vi "FGV_DataPackerParentVI.vi"(7 "Enum":T1, 10 "Callers (Main VI name)":string, 11 "This Computer Name":string) -> (2 "Parent VI to the DataPacker Daemon (Main VI name)":string, 3 "This Computer Name":string)   [LabVIEW 2018, in "feGEM DataPacker.lvlib"]
uses:
  Set_And_Get_Enum.ctl
  feGEM DataPacker.lvlib
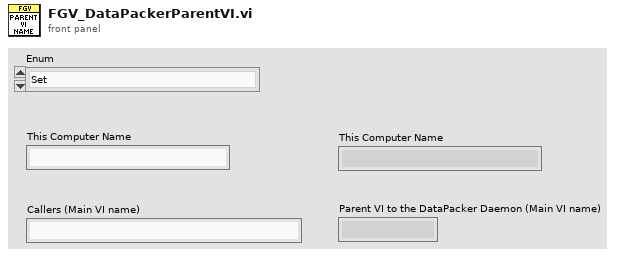
[diagram p1: front panel]
types:
  T1 = typedef "feGEM DataPacker.lvlib/Set_And_Get_Enum.ctl" = enum16{"Set", "Get"}
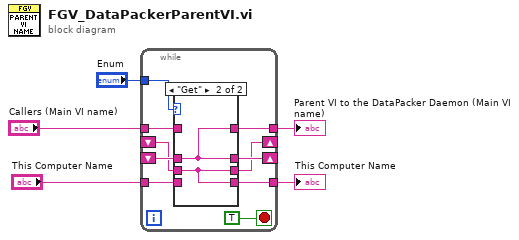
[diagram p0: block diagram]
diagram:
  n1 = while {
    tunnel: "Enum" -> [w15]
    tunnel: "Callers (Main VI name)" -> [w14]
    tunnel: [w13] -> w1
    shift-right: [w12] -> _
    shift-left: _ -> [w11]
    tunnel: "This Computer Name" -> [w9]
    tunnel: [w10] -> w2
    shift-right: [w8] -> _
    shift-left: _ -> [w7]
    stop <- TRUE stop-if-true
    n2 = case shown="\"Get\"" w15 {
      tunnel: w14 -> [w17 _]
      tunnel: [w17 w19] -> w13
      tunnel: [w17 w19] -> w12
      tunnel: w11 -> [_ w19]
      tunnel: [w16 w18] -> w10
      tunnel: w9 -> [w16 _]
      tunnel: [w16 w18] -> w8
      tunnel: w7 -> [_ w18]
      frame "Set", Default {
      }
      frame "Get" {
      }
    }
  }
  "This Computer Name" <- w2
  "Parent VI to the DataPacker Daemon (Main VI name)" <- w1
